vi "Read Name.vi"(7 "Linked List ID":string, 8 "error in (no error)":errorcluster, 11 "Linked List Ref":refnum<data-value>) -> (0 "error out":errorcluster, 2 "Header Value":string, 3 "Linked List Ref out":refnum<data-value>)   [LabVIEW 2019, in "Linked Lists.lvlib" / "Linked List Ref.lvclass"]
uses:
  <vilib>/gpm_packages/@cs/linked-list/Source/Linked List/Linked List Ref/Linked List Ref.lvclass
  <vilib>/gpm_packages/@cs/linked-list/Source/Linked List/ILinkedList/ILinked List.lvclass
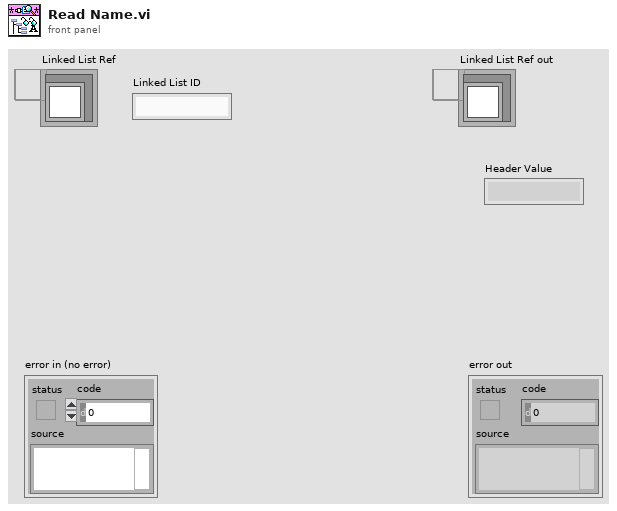
[diagram p1: front panel]
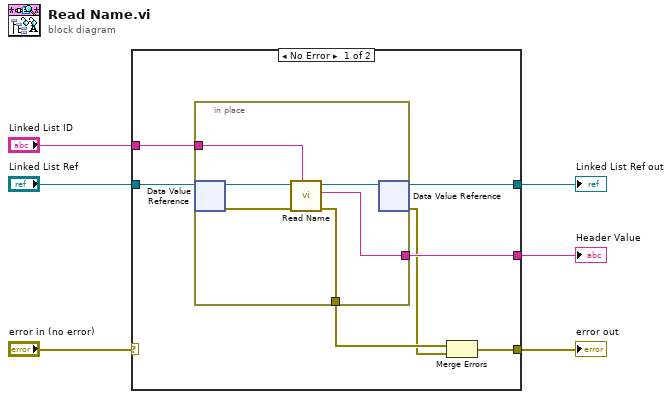
[diagram p0: block diagram]
diagram:
  n1 = case shown="No Error" "error in (no error)" {
    selector: "error in (no error)" -> [_ w21]
    tunnel: "Linked List Ref" -> [w13 w20]
    tunnel: "Linked List ID" -> [w12 _]
    tunnel: [w10 w21] -> w3
    tunnel: [w11 w20] -> w2
    tunnel: [w8 _] -> w1
    frame No Error {
      n2 = in-place {
        in-place-border: w12 -> [w17]
        in-place-border: [w15] -> w9
        in-place-border: [w14] -> w8
        n3 = in-place-dvr #1(w13) -> (w19:refnum<class "ILinked List.lvclass">, w16:errorcluster)
        n4 = call-dynamic "Read Name.vi"("Linked List ID"=w17, "error in (no error)"=w16, "ILinked List in"=w19) -> ("error out"=w15:errorcluster, "Name"=w14:string, "ILinked List out"=w18:refnum<class "ILinked List.lvclass">)  [unwired: 6 in]
        n5 = in-place-dvr #1(w18) -> (w11:refnum<data-value>, w7:errorcluster)
      }
      n6 = Merge Errors(w9, w7) -> (w10:errorcluster)
    }
    frame Error {
    }
  }
  "error out" <- w3
  "Linked List Ref out" <- w2
  "Header Value" <- w1
